vi "test DMM.vi"() -> ()   [LabVIEW 2013]
panel:
  in  "Boolean":bool
  in  "write buffer 2":string="read?"
  out "return count":u32=8
  in  "write buffer":string="rout:func 3\n"
  out "read buffer":string="SCAN OK\n"
  # "*idn?"
  # "conf:volt:dc"
  # "rout:del?"
  # "trig:coun_100"
  # "rout:mult:stat?"
  # "conf:curr:dc 0.5"
  # "val1?"
  # "read?"
  # "trig:sour_int   外部触发"
  # "rout:mult:open 117,117"
  # "rout:mult:clos"
  # "syst:loc"
  # "rout:coun 16  设置一次扫描启动channel个数"
  # "syst:rem"
  # "rout:func 3   开始SCAN"
  # "rout:func?"
  # "rout:func 0  放弃扫描"
  # "trig:auto_1"
  # "rout:open:all"
  # "trac:data?"
  # "rout:mult:open 115,116"
  # "rout:chan 101, 1, 2, 0"
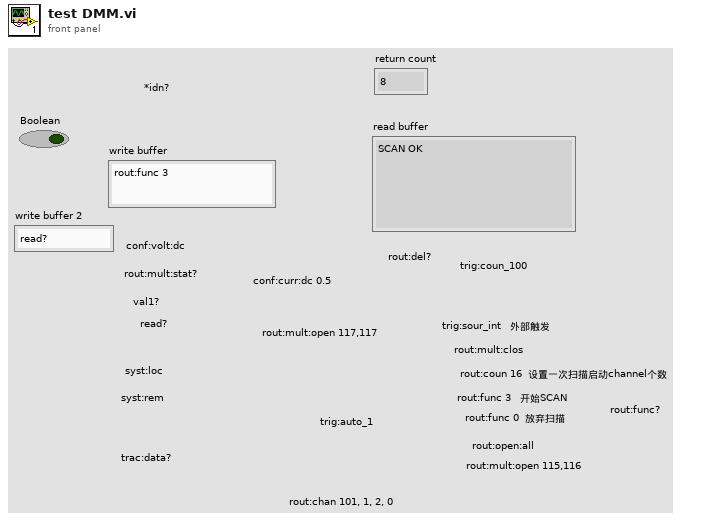
[diagram p1: front panel]
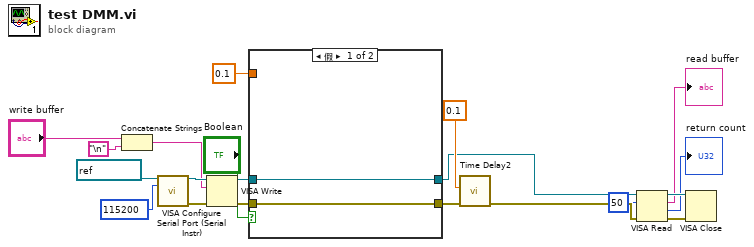
[diagram p0: block diagram]
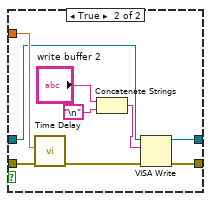
[diagram p2: hidden frame]
diagram:
  n1 = Concatenate Strings("write buffer", "\n") -> (w11:string)
  n2 = call <vilib>:"VISA Configure Serial Port (Serial Instr).vi"("VISA resource name"=refnum<visa-resource-name> "COM5", "baud rate (9600)"=u32 115200) -> ("VISA resource name out"=w18:refnum<visa-resource-name>, "error out"=w19:errorcluster)  [unwired: 12 in]
  n3 = VISA Write(VISA resource name=w18, write buffer=w11, error in (no error)=w19) -> (VISA resource name out=w8:refnum<visa-resource-name>, error out=w17:errorcluster)  [unwired: 1 out]
  n4 = case shown="假" "Boolean" {
    tunnel: 0.1 ("Delay Time (s)") -> [_ w31]
    tunnel: w17 -> [w22 w30]
    tunnel: w8 -> [w21 w28]
    tunnel: [w21 w27] -> w4
    tunnel: [w22 w26] -> w7
    frame False {
    }
    frame True {
      n5 = call "Time Delay"("error in (no error)"=w30, "Delay Time (s)"=w31) -> ("error out"=w29:errorcluster)  [unwired: 9 in]
      n6 = Concatenate Strings("write buffer 2", "\n") -> (w23:string)
      n7 = VISA Write(VISA resource name=w28, write buffer=w23, error in (no error)=w29) -> (VISA resource name out=w27:refnum<visa-resource-name>, error out=w26:errorcluster)  [unwired: 1 out]
    }
  }
  n8 = call "Time Delay2"("error in (no error)"=w7, "Delay Time (s)"=0.1) -> ("error out"=w3:errorcluster)  [unwired: 9 in]
  n9 = VISA Read(VISA resource name=w4, byte count=u32 50, error in (no error)=w3) -> (VISA resource name out=w15:refnum<visa-resource-name>, read buffer=→"read buffer":string, return count=→"return count":u32, error out=w16:errorcluster)
  n10 = VISA Close(VISA resource name=w15, error in (no error)=w16) -> ()  [unwired: 1 out]
